vi "Create Mesh Grid (2D).vi"   [LabVIEW 2024, in "NI_Gmath.lvlib"]
doc: "<p>Takes two <strong>x domain</strong> and <strong>y domain</strong> arrays and forms <strong>X</strong> and <strong>Y</strong> 2D arrays, which are typically used to evaluate and plot functions of two variables. You must <a href=\"nihelplauncher://docs/csh?context=lvcore_lvhowto_selectingdefaultinstpolyvi\">manually select the polymorphic instance</a> to use.</p>"
uses:
  NI_Gmath.lvlib
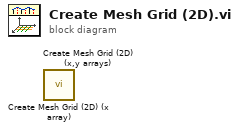
[diagram p0: block diagram]
diagram:
  n1 = call "Create Mesh Grid (2D) (x array).vi"() -> ()  [unwired: 9 in, 3 out]
  n2 = call "Create Mesh Grid (2D) (x,y arrays).vi"() -> ()  [unwired: 9 in, 3 out]
